vi "GenCtrl.vi"(6 "Loop Time (s)":dbl, 7 "Gen Control":T1, 8 "error in (no error)":errorcluster, 9 "ROSCO Params in":T6, 10 "IO Signals In":T5, 11 "ArrayPairs In":T3={"iStatus"={"Index"=0, "Value"=0.0}, "TIME"={"Index"=1, "Value"=0.0}, "DT"={"Index"=2, "Value"=0.0}, "Blade1PitchPos_rad"={"Index"=3, "Value"=0.0}, "VS_MECHGENPWR"={"Index"=13, "Value"=0.0}, "VS_GENPWR"={"Index"=14, "Value"=0.0}, "GEN_SPEED"={"Index"=19, "Value"=0.0}, "ROTOR_SPEED"={"Index"=20, "Value"=0.0}, "GENTQMEAS"={"Index"=22, "Value"=0.0}, "Y_M"={"Index"=23, "Value"=0.0}, "HORWINDV"={"Index"=26, "Value"=0.0}, "ROOTMOOP1"={"Index"=29, "Value"=0.0}, "ROOTMOOP2"={"Index"=30, "Value"=0.0}, "Blade2PitchPos_rad"={"Index"=32, "Value"=0.0}, "Blade3PitchPos_rad"={"Index"=33, "Value"=0.0}, "ROOTMOOP3"={"Index"=31, "Value"=0.0}, "AVCMSG_SIZE"={"Index"=48, "Value"=0.0}, "INFILE_SIZE "={"Index"=49, "Value"=0.0}, "OUTFILE_SIZE "={"Index"=50, "Value"=0.0}, "FA_ACC"={"Index"=52, "Value"=0.0}, "NUM_BLADES"={"Index"=60, "Value"=0.0}, "BladePitchSetpoint_rad"={"Index"=44, "Value"=0.0}, "TorqueSetpoint_Nm"={"Index"=46, "Value"=0.0}, "OUT_AEROTQ"={"Index"=89, "Value"=0.0}, "Out.RotSpeed "={"Index"=92, "Value"=0.0}, "Out.DEBUG"={"Index"=93, "Value"=0.0}}) -> (0 "error out":errorcluster, 1 "ROSCO Params Out":T6, 2 "IO Signals Out":T5, 3 "ArrayPairs Out":T3={"iStatus"={"Index"=0, "Value"=0.0}, "TIME"={"Index"=1, "Value"=0.0}, "DT"={"Index"=2, "Value"=0.0}, "Blade1PitchPos_rad"={"Index"=3, "Value"=0.0}, "VS_MECHGENPWR"={"Index"=13, "Value"=0.0}, "VS_GENPWR"={"Index"=14, "Value"=0.0}, "GEN_SPEED"={"Index"=19, "Value"=0.0}, "ROTOR_SPEED"={"Index"=20, "Value"=0.0}, "GENTQMEAS"={"Index"=22, "Value"=0.0}, "Y_M"={"Index"=23, "Value"=0.0}, "HORWINDV"={"Index"=26, "Value"=0.0}, "ROOTMOOP1"={"Index"=29, "Value"=0.0}, "ROOTMOOP2"={"Index"=30, "Value"=0.0}, "Blade2PitchPos_rad"={"Index"=32, "Value"=0.0}, "Blade3PitchPos_rad"={"Index"=33, "Value"=0.0}, "ROOTMOOP3"={"Index"=31, "Value"=0.0}, "AVCMSG_SIZE"={"Index"=48, "Value"=0.0}, "INFILE_SIZE "={"Index"=49, "Value"=0.0}, "OUTFILE_SIZE "={"Index"=50, "Value"=0.0}, "FA_ACC"={"Index"=52, "Value"=0.0}, "NUM_BLADES"={"Index"=60, "Value"=0.0}, "BladePitchSetpoint_rad"={"Index"=44, "Value"=0.0}, "TorqueSetpoint_Nm"={"Index"=46, "Value"=0.0}, "OUT_AEROTQ"={"Index"=89, "Value"=0.0}, "Out.RotSpeed "={"Index"=92, "Value"=0.0}, "Out.DEBUG"={"Index"=93, "Value"=0.0}}, 4 "Velocity setpoint (rad/s)":dbl, 5 "Torque setpoint (Nm)":dbl)   [LabVIEW 2018]
uses:
  Clusters/RoscoParams.ctl
  Clusters/IOSignals.ctl
  Clusters/ArrayPairs.ctl
  Clusters/SwapArrayCluster.ctl
  Clusters/GenCtrl.ctl
  Clusters/GenMode.ctl
  Clusters/GenCtrlMode.ctl
  <vilib>/addons/control/pid/pid.llb/PID Output Rate Limiter (DBL).vi
  <vilib>/addons/control/pid/NI_PID_pid.lvlib
panel:
  out "Current ramp time (s)":dbl
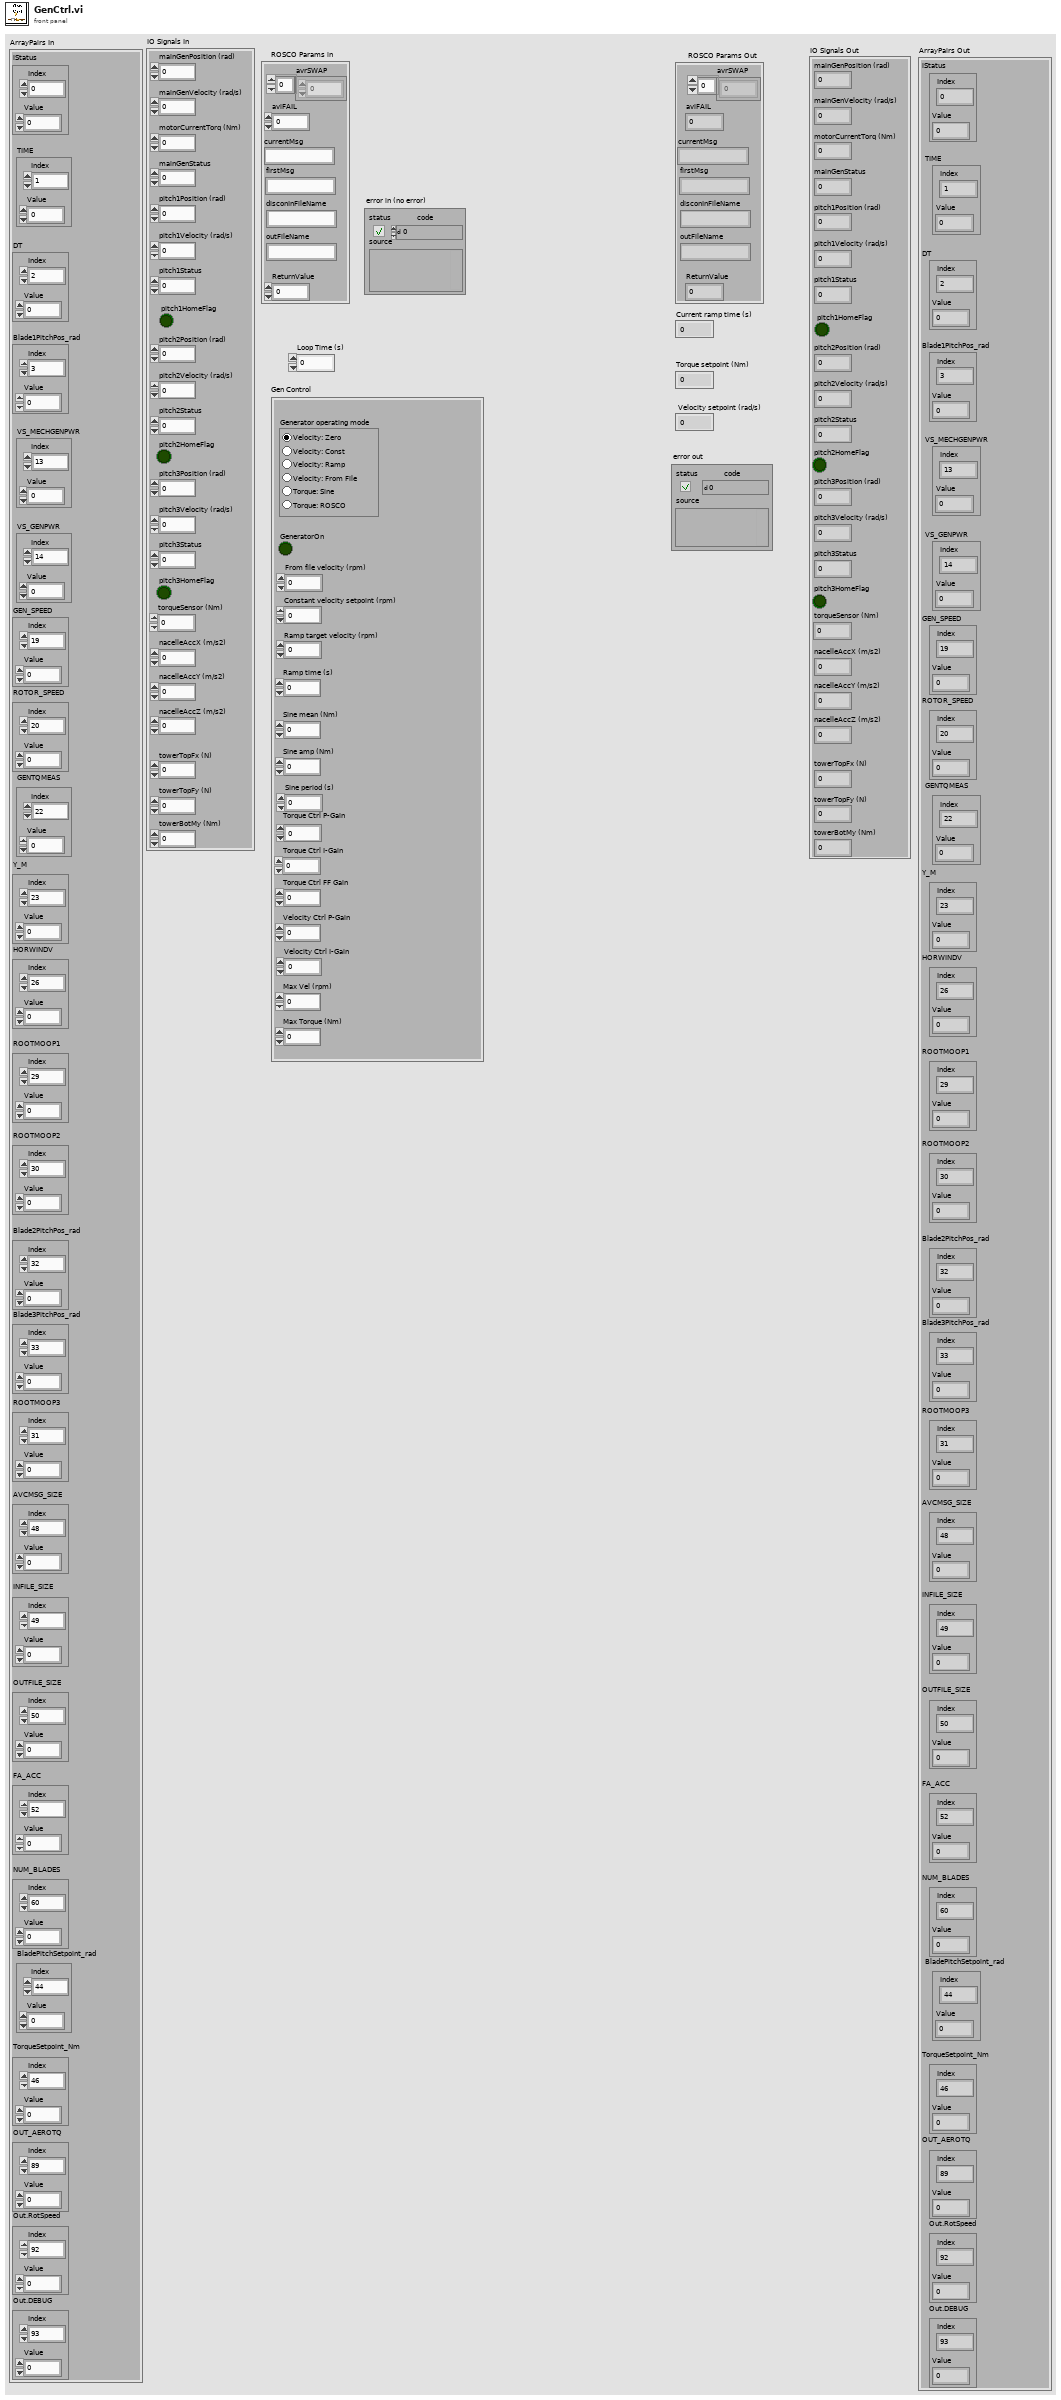
[diagram p1: front panel]
types:
  T1 = typedef "GenCtrl.ctl" = cluster{"Constant velocity setpoint (rpm)":dbl, "Ramp target velocity (rpm)":dbl, "Ramp time (s)":dbl, "Sine mean (Nm)":dbl, "Sine amp (Nm)":dbl, "Sine period (s)":dbl, "Torque Ctrl I-Gain":dbl, "Velocity Ctrl P-Gain":dbl, "Velocity Ctrl I-Gain":dbl, "Max Torque (Nm)":dbl, "GeneratorOn":bool, "Torque Ctrl P-Gain":dbl, "From file velocity (rpm)":dbl, "Generator operating mode":T2, "Max Vel (rpm)":dbl, "Torque Ctrl FF Gain":dbl}
  T2 = typedef "GenMode.ctl" = enum32{"Velocity: Zero", "Velocity: Const.", "Velocity: Ramp", "Velocity: From File", "Torque: Sine", "Torque: ROSCO"}
  T3 = typedef "ArrayPairs.ctl" = cluster{"iStatus":T4, "TIME":T4, "DT":T4, "Blade1PitchPos_rad":T4, "VS_MECHGENPWR":T4, "VS_GENPWR":T4, "GEN_SPEED":T4, "ROTOR_SPEED":T4, "GENTQMEAS":T4, "Y_M":T4, "HORWINDV":T4, "ROOTMOOP1":T4, "ROOTMOOP2":T4, "Blade2PitchPos_rad":T4, "Blade3PitchPos_rad":T4, "ROOTMOOP3":T4, "AVCMSG_SIZE":T4, "INFILE_SIZE ":T4, "OUTFILE_SIZE ":T4, "FA_ACC":T4, "NUM_BLADES":T4, "BladePitchSetpoint_rad":T4, "TorqueSetpoint_Nm":T4, "OUT_AEROTQ":T4, "Out.RotSpeed ":T4, "Out.DEBUG":T4}
  T4 = typedef "SwapArrayCluster.ctl" = cluster{"Index":i32, "Value":dbl}
  T5 = typedef "IOSignals.ctl" = cluster{"mainGenPosition (rad)":dbl, "motorCurrentTorq (Nm)":dbl, "mainGenVelocity (rad/s)":dbl, "mainGenStatus":u16, "pitch1Position (rad)":dbl, "pitch1Velocity (rad/s)":dbl, "pitch1Status":u16, "pitch2Position (rad)":dbl, "pitch2Velocity (rad/s)":dbl, "pitch2Status":u16, "pitch3Position (rad)":dbl, "pitch3Velocity (rad/s)":dbl, "pitch3Status":u16, "torqueSensor (Nm)":dbl, "nacelleAccX (m/s2)":dbl, "nacelleAccY (m/s2)":dbl, "nacelleAccZ (m/s2)":dbl, "pitch1HomeFlag":bool, "pitch2HomeFlag":bool, "pitch3HomeFlag":bool, "towerTopFx (N)":dbl, "towerTopFy (N)":dbl, "towerBotMy (Nm)":dbl}
  T6 = typedef "RoscoParams.ctl" = cluster{"avrSWAP":dbl[], "aviFAIL":i32, "currentMsg":string, "ReturnValue":i32, "disconInFileName":string, "outFileName":string, "firstMsg":string}
  T7 = typedef "GenCtrlMode.ctl" = enum16{"Torque Control", "Velocity Control"}
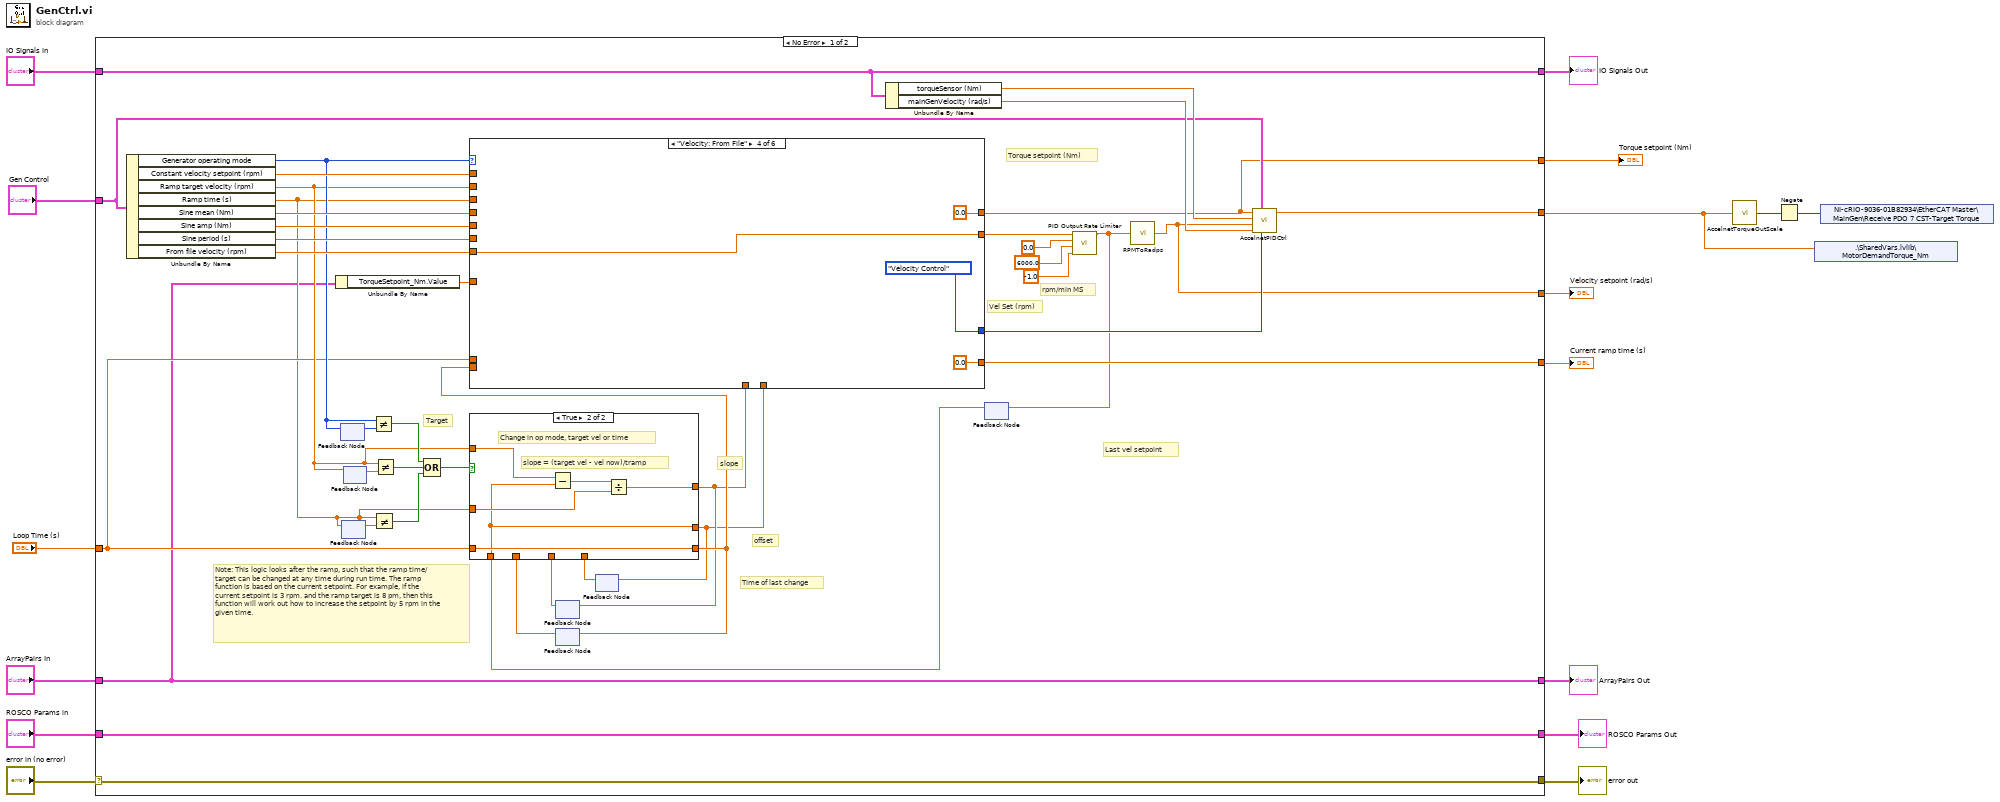
[diagram p0: block diagram]
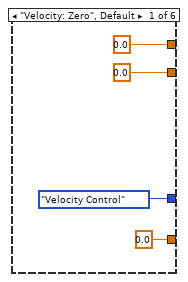
[diagram p3: hidden frame]
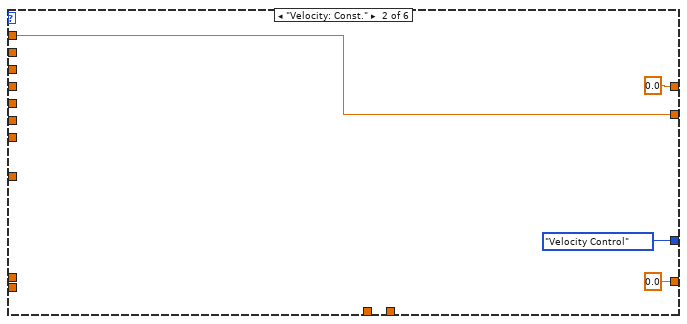
[diagram p4: hidden frame]
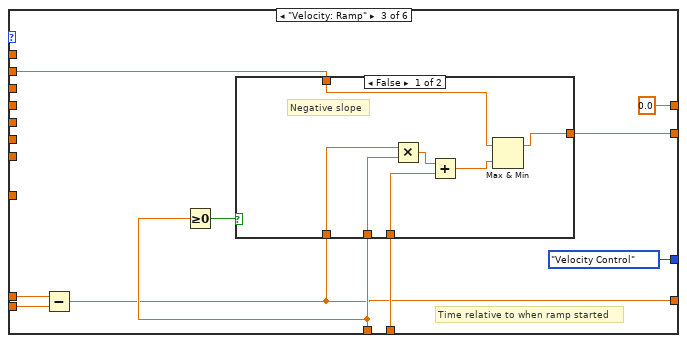
[diagram p5: hidden frame]
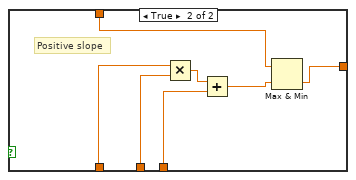
[diagram p6: hidden frame]
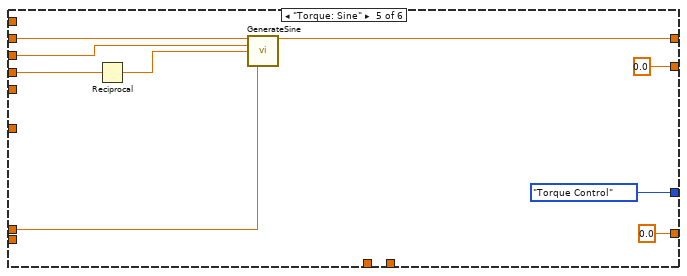
[diagram p7: hidden frame]
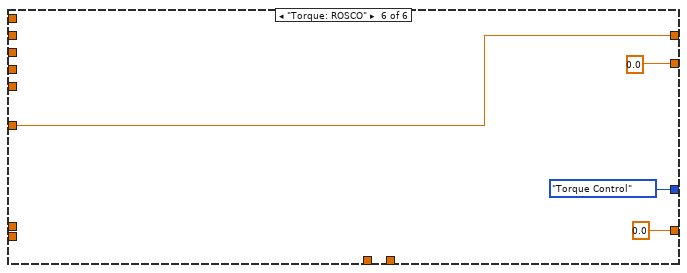
[diagram p8: hidden frame]
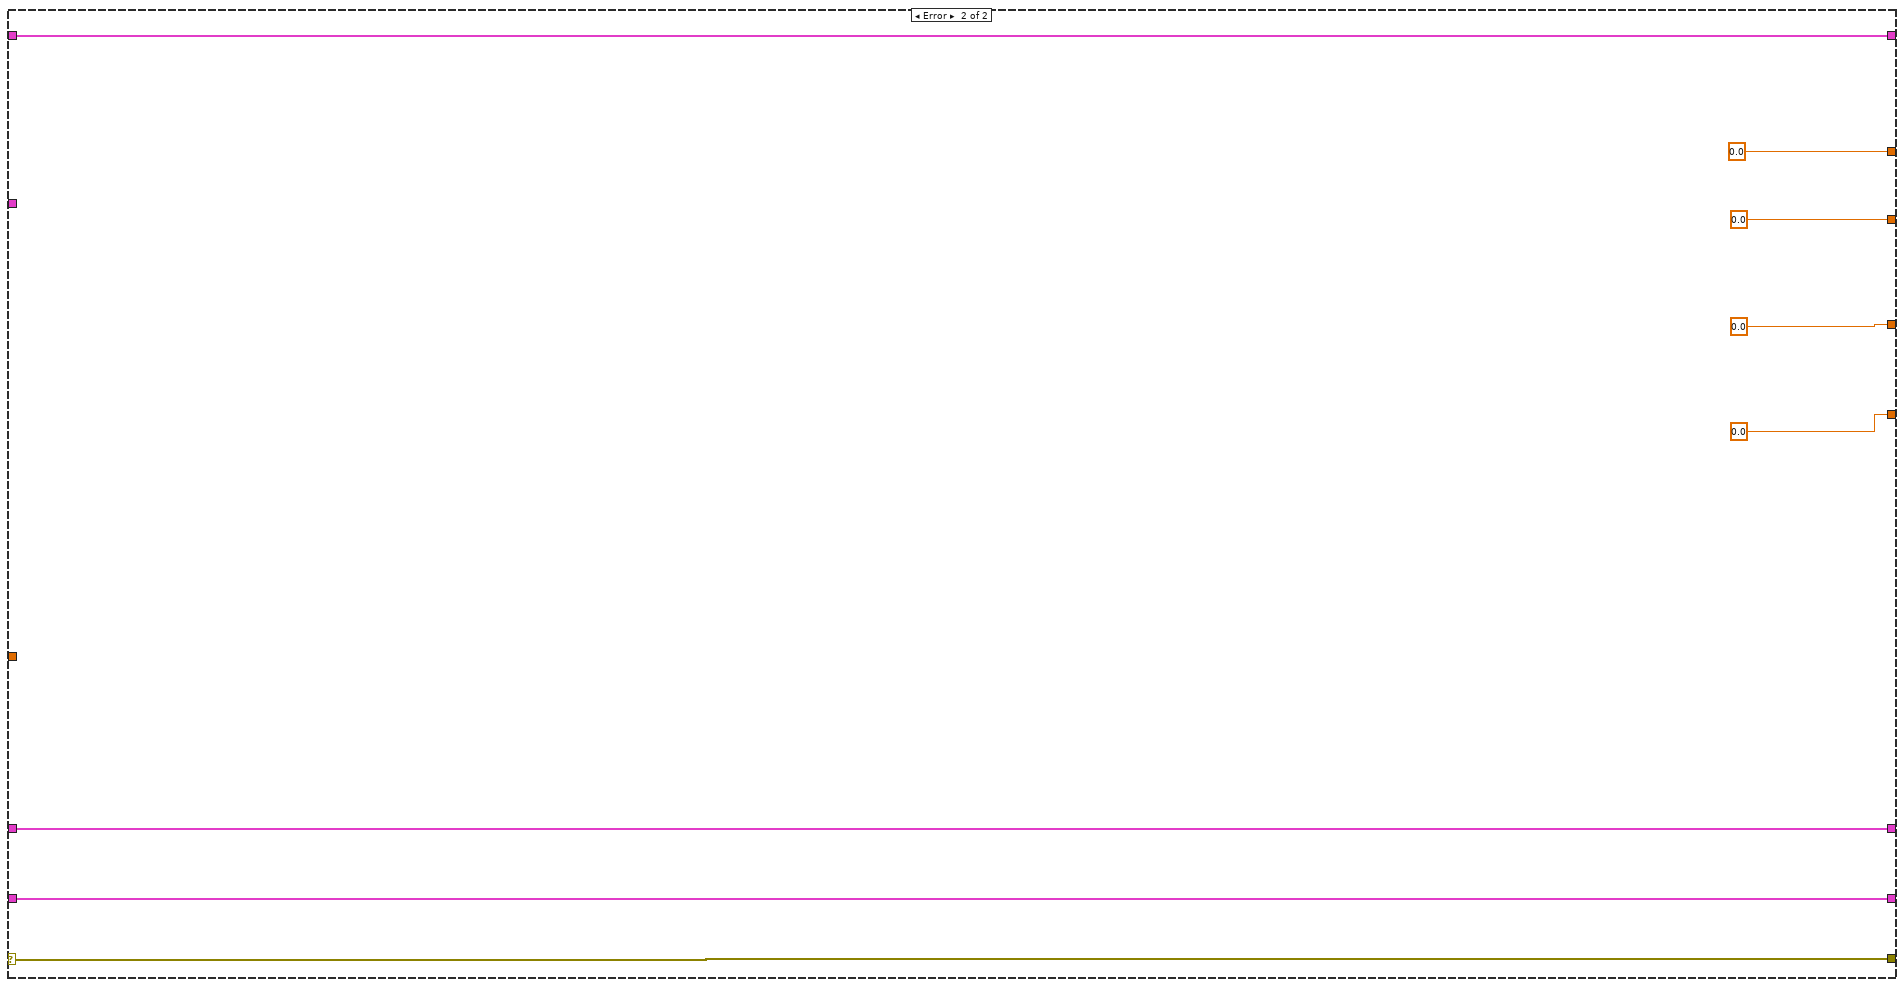
[diagram p9: hidden frame]
diagram:
  n1 = case shown="No Error" "error in (no error)" {
    selector: "error in (no error)" -> [w56 w123]
    tunnel: [w56 w123] -> w15
    tunnel: [w57 w122] -> w13
    tunnel: "ROSCO Params in" -> [w57 w122]
    tunnel: [w23 w121] -> w11
    tunnel: "ArrayPairs In" -> [w23 w121]
    tunnel: [w53 w120] -> w9
    tunnel: "IO Signals In" -> [w53 w120]
    tunnel: "Loop Time (s)" -> [w32 _]
    tunnel: "Gen Control" -> [w45 _]
    tunnel: [w54 0.0 ("Loop Time (s)")] -> w4
    tunnel: [w46 0.0] -> w2
    tunnel: [w26 0.0 ("Constant velocity setpoint (rpm)")] -> w6
    tunnel: [w44 0.0 ("Constant velocity setpoint (rpm)")] -> w5
    frame No Error {
      # "rpm/min MS"
      # "Note: This logic looks after the ramp, such that the ramp time/target can be changed at any time during run time. The ramp function is based on the current setpoint. For example, if the current setpoint is 3 rpm. and the ramp target is 8 pm, then this function will work out how to increase the setpoint by 5 rpm in the given time."
      # "offset"
      # "slope"
      # "Last vel setpoint"
      # "Time of last change"
      # "Target"
      # "Vel Set (rpm)"
      # "Torque setpoint (Nm)"
      n2 = Unbundle By Name(w45) -> ("Generator operating mode"=w42:T2, "Constant velocity setpoint (rpm)"=w55:dbl, "Ramp target velocity (rpm)"=w34:dbl, "Ramp time (s)"=w30:dbl, "Sine mean (Nm)"=w52:dbl, "Sine amp (Nm)"=w51:dbl, "Sine period (s)"=w50:dbl, "From file velocity (rpm)"=w43:dbl)
      n3 = Unbundle By Name(w23) -> ("TorqueSetpoint_Nm.Value"=w22:dbl)
      n4 = feedback-in #1(w42) -> ()
      n5 = feedback #1() -> (w41:T2)  [unwired: 1 in]
      n6 = feedback #2() -> (w39:dbl)  [unwired: 1 in]
      n7 = feedback-in #2(w30) -> ()
      n8 = feedback #3() -> (w40:dbl)  [unwired: 1 in]
      n9 = feedback-in #3(w34) -> ()
      n10 = Not Equal?(x=w42, y=w41) -> (x != y?=w36:bool)
      n11 = Not Equal?(x=w30, y=w39) -> (x != y?=w38:bool)
      n12 = Not Equal?(x=w34, y=w40) -> (x != y?=w37:bool)
      n13 = Compound Arithmetic op=OR(w36, w37, w38) -> (w35:bool)
      n14 = feedback #4() -> (w28:dbl)  [unwired: 1 in]
      n15 = feedback #5() -> (w33:dbl)  [unwired: 1 in]
      n16 = feedback #6() -> (w24:dbl)  [unwired: 1 in]
      n17 = Unbundle By Name(w53) -> ("torqueSensor (Nm)"=w49:dbl, "mainGenVelocity (rad/s)"=w48:dbl)
      n18 = feedback #7() -> (w27:dbl)  [unwired: 1 in]
      n19 = case shown="True" w35 {
        tunnel: w27 -> [_ w61]
        tunnel: w34 -> [_ w65]
        tunnel: w32 -> [_ w66]
        tunnel: [w60 w66] -> w31
        tunnel: w33 -> [w60 _]
        tunnel: w30 -> [_ w63]
        tunnel: [w59 w62] -> w29
        tunnel: w28 -> [w59 _]
        tunnel: [w58 w61] -> w25
        tunnel: w24 -> [w58 _]
        frame False {
        }
        frame True {
          # "slope = (target vel - vel now)/tramp"
          # "Change in op mode, target vel or time"
          n20 = Subtract(x=w65, y=w61) -> (x-y=w64:dbl)
          n21 = Divide(x=w64, y=w63) -> (x/y=w62:dbl)
        }
      }
      n22 = case shown="\"Velocity: From File\"" w42 {
        tunnel: w55 -> [_ w71 _ _ _ _]
        tunnel: w34 -> [_ _ w76 _ _ _]
        tunnel: w30 -> [_ _ _ _ _ _]
        tunnel: [0.0 ("Constant velocity setpoint (rpm)") 0.0 ("Constant velocity setpoint (rpm)") w77 0.0 ("Constant velocity setpoint (rpm)") 0.0 ("Constant velocity setpoint (rpm)") 0.0 ("Constant velocity setpoint (rpm)")] -> w54
        tunnel: w52 -> [_ _ _ _ w110 _]
        tunnel: [0.0 ("Constant velocity setpoint (rpm)") 0.0 ("Constant velocity setpoint (rpm)") 0.0 ("Constant torque setpoint (Nm)") 0.0 ("Constant torque setpoint (Nm)") w103 w112] -> w44
        tunnel: w51 -> [_ _ _ _ w109 _]
        tunnel: w50 -> [_ _ _ _ w108 _]
        tunnel: [0.0 ("Constant velocity setpoint (rpm)") w71 w75 w99 0.0 ("Constant velocity setpoint (rpm)") 0.0 ("Constant velocity setpoint (rpm)")] -> w18
        tunnel: [GenCtrlMode."Velocity Control" GenCtrlMode."Velocity Control" GenCtrlMode."Velocity Control" GenCtrlMode."Velocity Control" GenCtrlMode."Torque Control" GenCtrlMode."Torque Control"] -> w47
        tunnel: w43 -> [_ _ _ w99 _ _]
        tunnel: w32 -> [_ _ w82 _ w104 _]
        tunnel: w31 -> [_ _ w81 _ _ _]
        tunnel: w29 -> [_ _ w78 _ _ _]
        tunnel: w25 -> [_ _ w79 _ _ _]
        tunnel: w22 -> [_ _ _ _ _ w112]
        frame "Velocity: Zero", Default {
        }
        frame "Velocity: Const." {
        }
        frame "Velocity: Ramp" {
          # "Time relative to when ramp started"
          n23 = Subtract(x=w82, y=w81) -> (x-y=w77:dbl)
          n24 = Greater Or Equal To 0?(x=w78) -> (x >= 0?=w80:bool)
          n25 = case shown="False" w80 {
            tunnel: w79 -> [w88 w95]
            tunnel: w78 -> [w90 w96]
            tunnel: w77 -> [w91 w97]
            tunnel: w76 -> [w86 w93]
            tunnel: [w85 w92] -> w75
            frame False {
              # "Negative slope"
              n26 = Multiply(x=w91, y=w90) -> (x*y=w89:dbl)
              n27 = Add(x=w89, y=w88) -> (x+y=w87:dbl)
              n28 = Max & Min(x=w86, y=w87) -> (max(x,y)=w85:dbl)  [unwired: 1 out]
            }
            frame True {
              # "Positive slope"
              n29 = Multiply(x=w97, y=w96) -> (x*y=w98:dbl)
              n30 = Add(x=w98, y=w95) -> (x+y=w94:dbl)
              n31 = Max & Min(x=w93, y=w94) -> (min(x,y)=w92:dbl)  [unwired: 1 out]
            }
          }
        }
        frame "Velocity: From File" {
        }
        frame "Torque: Sine" {
          n32 = Reciprocal(x=w108) -> (1/x=w107:dbl)
          n33 = call "GenerateSine.vi"("Mean"=w110, "Amplitude"=w109, "frequency (f)"=w107, "time (s)"=w104) -> ("sine out"=w103:dbl)  [unwired: 11 in]
        }
        frame "Torque: ROSCO" {
        }
      }
      n34 = feedback-in #4(w29) -> ()
      n35 = feedback-in #5(w31) -> ()
      n36 = feedback-in #6(w25) -> ()
      n37 = call-poly <vilib>:"PID Output Rate Limiter.vi"("dt (s)"=-1.0, "output rate (EGU/min)"=6000.0, "initial output"=0.0, "input (controller output)"=w18) -> ("output"=w17:dbl)  [unwired: 4 in, 1 out]
      n38 = feedback-in #7(w17) -> ()
      n39 = call "RPMToRadps.vi"("rpm"=w17) -> ("rad/s"=w26:dbl)
      n40 = call "AccelnetPIDCtrl.vi"("Control Mode"=w47, "Gen Control"=w45, "Motor actual velocity (rad/s)"=w48, "Velocity setpoint (rad/s)"=w26, "Torque Sensor (Nm)"=w49, "Torque Setpoint (Nm)"=w44) -> ("Torque demand (Nm)"=w46:dbl)  [unwired: 5 in]
    }
    frame Error {
    }
  }
  "error out" <- w15
  "ROSCO Params Out" <- w13
  "IO Signals Out" <- w9
  "ArrayPairs Out" <- w11
  "Current ramp time (s)" <- w4
  "Torque setpoint (Nm)" <- w5
  "Velocity setpoint (rad/s)" <- w6
  n41 = call "AccelnetTorqueOutScale.vi"("Demand torque (Nm)"=w2) -> ("Torque setpoint to drive"=w3:i16)
  n42 = Negate(x=w3) -> (-x=w1:i16)
  n43 = shared-variable ".\\SharedVars.lvlib\\MotorDemandTorque_Nm"(w2) -> ()  [unwired: 1 in, 1 out]
  n44 = shared-variable "NI-cRIO-9036-01B82934\\EtherCAT Master\\MainGen\\Receive PDO 7 CST-Target Torque"(w1) -> ()  [unwired: 1 in, 1 out]
